vi "Configure Digital Signal Interface Module.vi"(6 "Loop Back Test (3: Device)":u16(ring)=3 items=["Digital Bus", "Cable", "N5102A", "Device"], 7 "Enable Digital Signal Interface Module (F:Disable)":bool, 8 "error in (no error)":errorcluster, 9 "Data Transmission Type (0: Parallel)":u16(ring) items=["Parallel", "Serial", "Parallel interleaving I/Q", "Parallel interleaving I"], 10 "Logic Data Type (5: 3.3 volt CMOS signal)":u16(ring)=5 items=["Low voltage differential signal", "Low voltage TTL signal", "1.5 volt CMOS signal", "1.8 volt CMOS signal", "2.5 volt CMOS signal", "3.3 volt CMOS signal"], 11 "VISA resource name":refnum<visa-resource-name>) -> (0 "error out":errorcluster, 3 "VISA resource name out":refnum<visa-resource-name>)   [LabVIEW 2012, in "Agilent PSG MXG Series.lvlib"]
doc: "Configures digital signal interface module N5102A.\n\n<B>Notes:</B>\n(1) This VI is valid only in E8267D that installs <B>Option 601</B> or <B>Option 602</B> (Internal baseband generator), and <B>Option 003</B> (PSG digital output connectivity with N5102A) or <B>Option 004</B> (PSG digital input connectivity with N5102A)."
uses:
  <instrlib>/Agilent PSG MXG Series/Agilent PSG MXG Series.lvlib
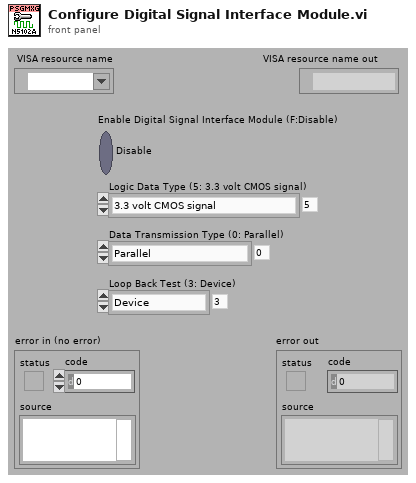
[diagram p1: front panel]
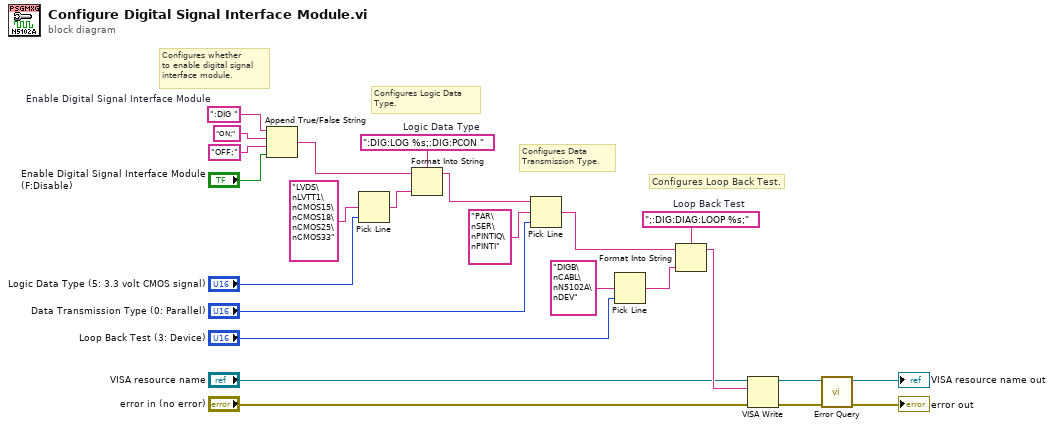
[diagram p0: block diagram]
diagram:
  w11 = ";:DIG:DIAG:LOOP %s;"  # Loop Back Test
  w18 = ":DIG:LOG %s;:DIG:PCON "  # Logic Data Type
  w24 = ":DIG "  # Enable Digital Signal Interface Module
  # "Configures Loop Back Test."
  # "Configures Data\nTransmission Type."
  # "Configures Logic Data\nType."
  # "Configures whether\nto enable digital signal\ninterface module."
  n1 = Append True/False String(1:"Enable Digital Signal Interface Module (F:Disable)", 2:"OFF;" ("false string"), 3:"ON;" ("true string"), 4:w24) -> (0:w19:string)
  n2 = Pick Line(multi-line string="LVDS\nLVTT1\nCMOS15\nCMOS18\nCMOS25\nCMOS33", line index="Logic Data Type (5: 3.3 volt CMOS signal)") -> (output string=w17:string)  [unwired: 1 out]
  n3 = Format Into String(format string=w18, initial string=w19, w17) -> (resulting string=w15:string)  [unwired: 1 in, 1 out]
  n4 = Pick Line(string ("")=w15, multi-line string="PAR\nSER\nPINTIQ\nPINTI", line index="Data Transmission Type (0: Parallel)") -> (output string=w12:string)
  n5 = Pick Line(multi-line string="DIGB\nCABL\nN5102A\nDEV", line index="Loop Back Test (3: Device)") -> (output string=w9:string)  [unwired: 1 out]
  n6 = Format Into String(format string=w11, initial string=w12, w9) -> (resulting string=w7:string)  [unwired: 1 in, 1 out]
  n7 = VISA Write(VISA resource name="VISA resource name", write buffer=w7, error in (no error)="error in (no error)") -> (VISA resource name out=w6:refnum<visa-resource-name>, error out=w5:errorcluster)  [unwired: 1 out]
  n8 = call <instrlib>:"Error Query.vi"("error in (no error)"=w5, "VISA resource name"=w6) -> ("error out"=→"error out":errorcluster, "VISA resource name out"=→"VISA resource name out":refnum<visa-resource-name>)  [unwired: 8 out]
